vi "Initialize by Serial.vi"(8 "error in (no error)":errorcluster, 11 "Serial Number":string) -> (0 "error out":errorcluster, 3 "device handle out":T1)   [LabVIEW 2021, in "RTL-SDR.lvlib"]
uses:
  RTL-SDR.lvlib
  usr/lib64/librtlsdr.so.0
  Controls/Device Handle.ctl
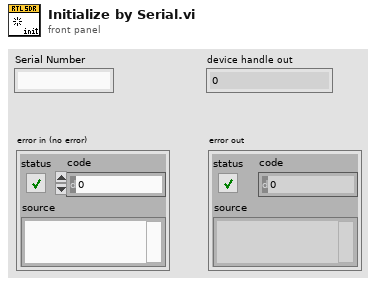
[diagram p1: front panel]
types:
  T1 = typedef "RTL-SDR.lvlib/Device Handle.ctl" = u64
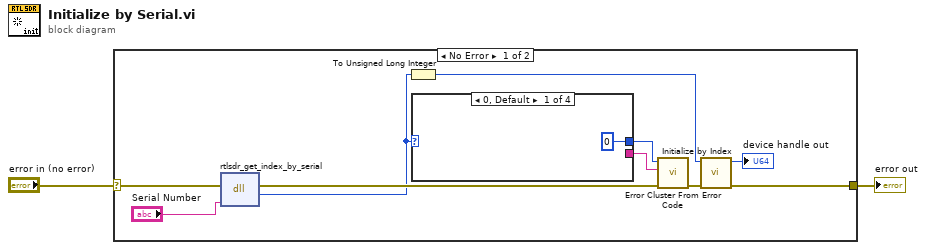
[diagram p0: block diagram]
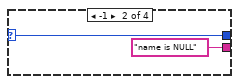
[diagram p2: hidden frame]
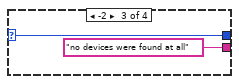
[diagram p3: hidden frame]
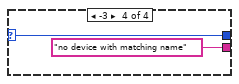
[diagram p4: hidden frame]
diagram:
  n1 = case shown="No Error" "error in (no error)" {
    selector: "error in (no error)" -> [w5 w20]
    tunnel: [w12 w20] -> w2
    frame No Error {
      n2 = dll-call lib="usr/lib64/librtlsdr.so.0" fn="rtlsdr_get_index_by_serial"(error in=w5, "serial"="Serial Number") -> (error out=w11:errorcluster, "index"=w9:i32)  [unwired: 3 in, 1 out]
      n3 = To Unsigned Long Integer(number=w9) -> (unsigned 32bit integer=w3:u32)
      n4 = case shown="0, Default" w9 {
        selector: w9 -> [_ w14 w17 w19]
        tunnel: [0 ("index") w14 w17 w19] -> w8
        tunnel: [_ "name is NULL" ("error message (\"\")") "no devices were found at all" ("error message (\"\")") "no device with matching name" ("error message (\"\")")] -> w7
        frame 0, Default {
        }
        frame -1 {
        }
        frame -2 {
        }
        frame -3 {
        }
      }
      n5 = call <vilib>:"Error Cluster From Error Code.vi"("error in (no error)"=w11, "error message (\"\")"=w7, "error code (0)"=w8) -> ("error out"=w10:errorcluster)  [unwired: 6 in]
      n6 = call "Initialize by Index.vi"("error in (no error)"=w10, "device index"=w3) -> ("error out"=w12:errorcluster, "device handle out"=→"device handle out":T1)  [unwired: 8 in]
    }
    frame Error {
    }
  }
  "error out" <- w2
